vi "1.数字IO节点使用.vi"   [LabVIEW 2019]
uses:
  <vilib>/rvi/Emulation/niFpgaGetClockAttributes.vi
  <vilib>/rvi/Emulation/niFpgaSctlEmulationGetInTimedLoop.vi
  <vilib>/rvi/Emulation/niFpgaEmulationReportErrorSimple.vi
  <vilib>/rvi/eio/common/nirviEmuTemplateMethod_errors.vi
  <vilib>/rvi/Emulation/niFpgaCriticalErrorInLSC.vi
  <vilib>/eio/EIONode/EIONode.xnode
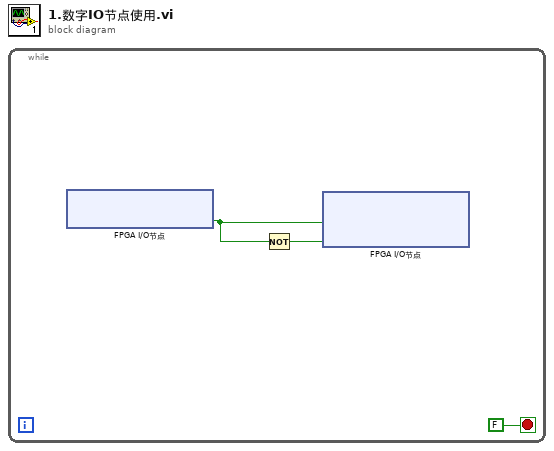
[diagram p0: block diagram]
diagram:
  n1 = while {
    stop <- FALSE stop-if-true
    n2 = xnode "FPGA I/O节点"() -> ("ConnectorA/DIO0"=w1:bool)  [unwired: 1 in, 1 out]
    n3 = Not(x=w1) -> (.not. x?=w2:bool)
    n4 = xnode "FPGA I/O节点"("ConnectorA/DIO2"=w1, "ConnectorA/DIO3"=w2) -> ()  [unwired: 2 in, 2 out]
  }
